vi "Mouse Up - Toggle Check Box.vi"(8 "error in (no error)":errorcluster, 10 "Coords":T1, 11 "MCListbox with Checkboxes in":refnum<class "MCListbox with Checkboxes.lvclass">) -> (0 "error out":errorcluster, 2 "In Check?":bool, 3 "MCListbox with Checkboxes out":refnum<class "MCListbox with Checkboxes.lvclass">)   [LabVIEW 2016, in "MCListbox with Checkboxes.lvclass"]
uses:
  MCListbox with Checkboxes.lvclass
  <vilib>/Utility/miscctls.llb/LVPoint32TypeDef.ctl
  MCListbox with Checkboxes.lvclass/MCListbox with Checkboxes.ctl
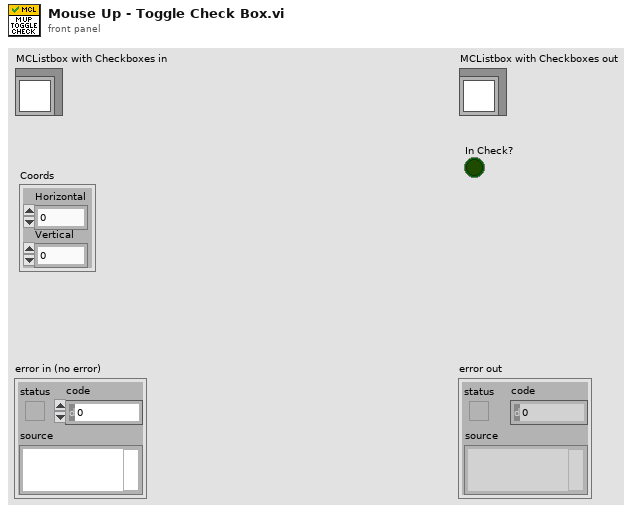
[diagram p1: front panel]
types:
  T1 = typedef "LVPoint32TypeDef.ctl" = cluster{"Horizontal":i32, "Vertical":i32}
  T2 = typedef "LVRowAndColumnTypeDef.ctl" = cluster{"Row":i32, "Column":i32}
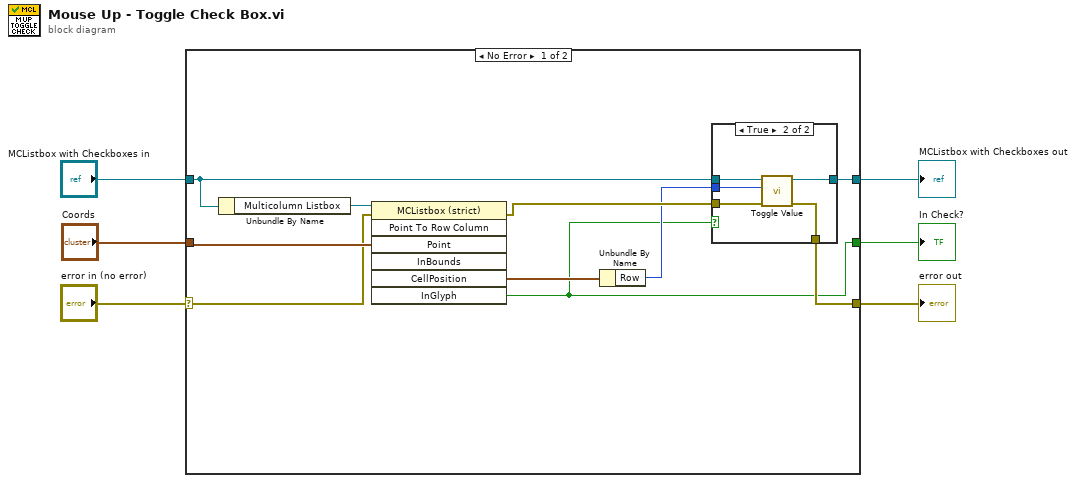
[diagram p0: block diagram]
diagram:
  n1 = case shown="No Error" "error in (no error)" {
    selector: "error in (no error)" -> [w9 w25]
    tunnel: [w15 w25] -> w5
    tunnel: [w16 w24] -> w4
    tunnel: "MCListbox with Checkboxes in" -> [w12 w24]
    tunnel: "Coords" -> [w13 _]
    tunnel: [w7 _] -> w2
    frame No Error {
      n2 = Unbundle By Name(w12) -> ("Multicolumn Listbox"=w14:refnum<vi>)
      n3 = invoke class="MCListbox (strict)" method="Point To Row Column"(reference=w14, error in=w9, "Point"=w13) -> (error out=w11:errorcluster, "CellPosition"=w10:T2, "InGlyph"=w7:bool)  [unwired: 4 in, 4 out]
      n4 = Unbundle By Name(w10) -> ("Row"=w8:i32)
      n5 = case shown="True" w7 {
        tunnel: [w18 w23] -> w16
        tunnel: [w17 w22] -> w15
        tunnel: w12 -> [w18 w21]
        tunnel: w11 -> [w17 w20]
        tunnel: w8 -> [_ w19]
        frame False {
        }
        frame True {
          n6 = call "Toggle Value.vi"("error in (no error)"=w20, "Index"=w19, "MCListbox with Checkboxes in"=w21) -> ("error out"=w22:errorcluster, "MCListbox with Checkboxes out"=w23:refnum<class "MCListbox with Checkboxes.lvclass">)  [unwired: 7 in]
        }
      }
    }
    frame Error {
    }
  }
  "error out" <- w5
  "MCListbox with Checkboxes out" <- w4
  "In Check?" <- w2
